vi "File_path.vi"(8 "error in (no error)":errorcluster, 10 "Direccion":path, 11 "GUI_Actor in":refnum<class "GUI_Actor.lvclass">) -> (0 "error out":errorcluster, 3 "GUI_Actor out":refnum<class "GUI_Actor.lvclass">)   [LabVIEW 2019, in "GUI_Actor.lvlib" / "GUI_Actor.lvclass"]
uses:
  GUI_Actor.lvclass
  GUI_Actor.lvclass/GUI_Actor.ctl
  Logging_txt/Logging_txt Messages/Write Direccion Msg/Write Direccion Msg.lvclass/Write Direccion Msg.ctl
  <vilib>/ActorFramework/Message Enqueuer/Message Enqueuer.lvclass/Message Enqueuer.ctl
  <vilib>/ActorFramework/Message Enqueuer/Enqueue.vi
  Logging_txt/Logging_txt Messages/Write Direccion Msg/Write Direccion Msg.lvclass
  C:/Program Files/National Instruments/LabVIEW 2019/vi.lib/ActorFramework/Message/Message.lvclass
  <vilib>/ActorFramework/Message Priority Queue/Priority Enqueue.vi
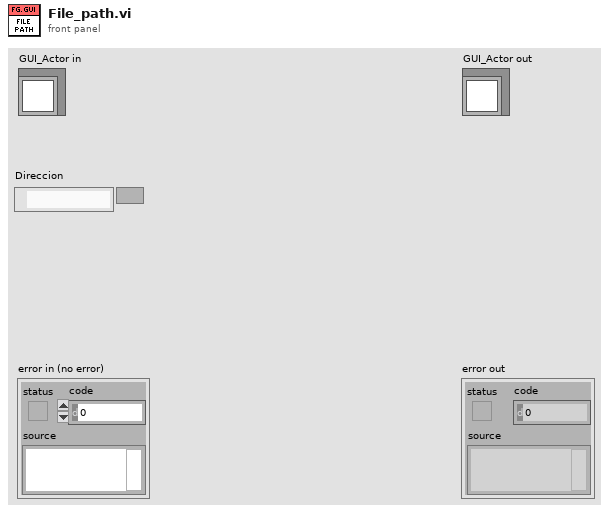
[diagram p1: front panel]
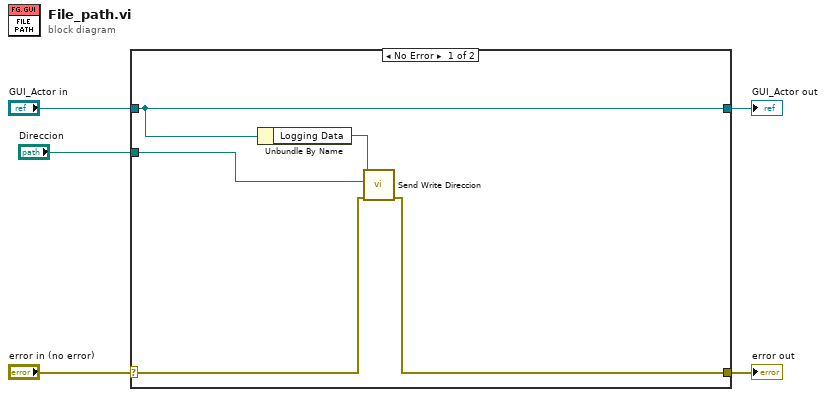
[diagram p0: block diagram]
diagram:
  n1 = case shown="No Error" "error in (no error)" {
    selector: "error in (no error)" -> [w7 w12]
    tunnel: [w6 w12] -> w4
    tunnel: [w9 w11] -> w2
    tunnel: "GUI_Actor in" -> [w9 w11]
    tunnel: "Direccion" -> [w10 _]
    frame No Error {
      n2 = Unbundle By Name(w9) -> ("Logging Data"=w8:refnum<class "Message Enqueuer.lvclass">)
      n3 = call "Send Write Direccion.vi"("error in (no error)"=w7, "Direccion"=w10, "Message Enqueuer"=w8) -> ("error out"=w6:errorcluster)  [unwired: 7 in, 1 out]
    }
    frame Error {
    }
  }
  "error out" <- w4
  "GUI_Actor out" <- w2
